vi "Modbus RT Driver VI Modbus.vi"(4 "DEBUG RT-FIFOs Indexes":T1[](array[typedef]), 6 "DEBUG General Settings":T3 {"Communication_Type" items=["TCP", "Serial"]; "Modbus_Type" items=["Master", "Slave"]; "Serial Settings"."Serial_Settings_Flow_Control" items=["None", "XONXOFF", "RTSCTS", "XONXOFFANDRTSCTS", "DTRDSR", "XONXOFFANDDTRDSR"]; "Serial Settings"."Serial_Settings_Parity" items=["None", "Odd", "Even"]; "Serial Settings"."Serial_Settings_Serial_Type" items=["RTU", "ASCII"]}, 7 "First FIFO Index of Status Channels":i32, 8 "error in (no error)":errorcluster, 9 "Inputs In":dbl[](array[numeric]), 10 "DEBUG Modbus Items":T9[](array[typedef]), 11 "Outputs In":dbl[](array[numeric])) -> (0 "error out":errorcluster, 3 "Outputs Out":dbl[](array[numeric]))   [LabVIEW 2014, in "Modbus Engine.lvlib"]
uses:
  Modbus Engine.lvlib
  XML Deserializer/XML VIs/API/Controls/Modbus_Items.ctl
  XML Deserializer/XML VIs/API/Controls/Modbus_Item_Type.ctl
  XML Deserializer/XML VIs/API/Controls/Modbus_General_Settings.ctl
  XML Deserializer/XML VIs/API/Controls/Modbus_Communication_Type.ctl
  XML Deserializer/XML VIs/API/Controls/Modbus_Type.ctl
  XML Deserializer/XML VIs/API/Controls/Modbus_Serial_Settings_Flow_Control.ctl
  XML Deserializer/XML VIs/API/Controls/Modbus_Serial_Settings_Parity.ctl
  XML Deserializer/XML VIs/API/Controls/Modbus_Serial_Settings_Serial_Type.ctl
  Shared/FIFO Indexes.ctl
  <vilib>/NI Veristand/Custom Device API/Custom Device Channel Type.ctl
  Modbus RT Driver VI States Definition.ctl
  ModbusPharLap.lvlibp/Modbus Library/API/Modbus API.lvclass
  <vilib>/NI Veristand/Custom Device Tools/Custom Device Utility Library/RT Debug String Color Spec.ctl
  Shared/Modbus Shared.lvlib
  ModbusPharLap.lvlibp/Modbus Library/API/Wrapper/API Main.lvlib
  <vilib>/NI Veristand/Custom Device Tools/Custom Device Utility Library/Custom Device Utility Library.lvlib
  ModbusPharLap.lvlibp/Modbus Library/API/Master/Modbus Master.lvclass
  <vilib>/NI Veristand/Custom Device API/Custom Device API.lvlib
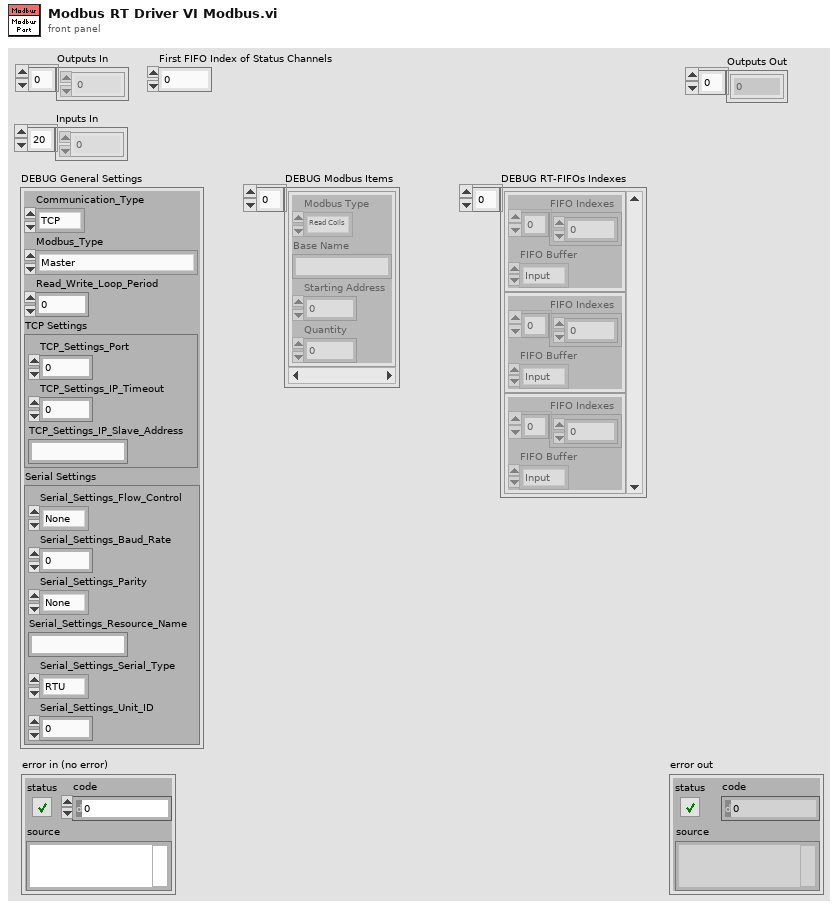
[diagram p1: front panel]
types:
  T1 = typedef "Modbus Shared.lvlib/FIFO Indexes.ctl" = cluster{"FIFO Indexes":i32[], "FIFO Buffer":T2}
  T2 = typedef "Custom Device API.lvlib/Custom Device Channel Type.ctl" = enum16{"Input", "Output"}
  T3 = typedef "Modbus Shared.lvlib/Modbus_General_Settings.ctl" = cluster{"Communication_Type":T4, "Modbus_Type":T5, "Read_Write_Loop_Period":i64, "TCP Settings":cluster{"TCP_Settings_Port":u16, "TCP_Settings_IP_Timeout":u32, "TCP_Settings_IP_Slave_Address":string}, "Serial Settings":cluster{"Serial_Settings_Flow_Control":T6, "Serial_Settings_Baud_Rate":u32, "Serial_Settings_Parity":T7, "Serial_Settings_Resource_Name":string, "Serial_Settings_Serial_Type":T8, "Serial_Settings_Unit_ID":u8}}
  T4 = typedef "Modbus Shared.lvlib/Modbus_Communication_Type.ctl" = i32
  T5 = typedef "Modbus Shared.lvlib/Modbus_Type.ctl" = i32
  T6 = typedef "Modbus Shared.lvlib/Modbus_Serial_Settings_Flow_Control.ctl" = i32
  T7 = typedef "Modbus Shared.lvlib/Modbus_Serial_Settings_Parity.ctl" = i32
  T8 = typedef "Modbus Shared.lvlib/Modbus_Serial_Settings_Serial_Type.ctl" = i32
  T9 = typedef "Modbus Shared.lvlib/Modbus_Items.ctl" = cluster{"Modbus Type":T10, "Base Name":string, "Starting Address":u16, "Quantity":u16}
  T10 = typedef "Modbus Shared.lvlib/Modbus_Item_Type.ctl" = enum16{"Read Coils", "Read Discrete Inputs", "Read Holding Registers", "Read Input Registers", "Write Multiple Coils", "Write Multiple Holding Registers", "Write Single Coil", "Write Single Holding Register", "Write Multiple Discrete Inputs", "Write Multiple Input Registers"}
  T11 = typedef "Modbus Engine.lvlib/Modbus RT Driver VI States Definition.ctl" = enum16{"Initialization", "Master - Connect", "Slave - Create Instance", "Exit", "Connected"}
  T12 = typedef "Custom Device Utility Library.lvlib/RT Debug String Color Spec.ctl" = u16
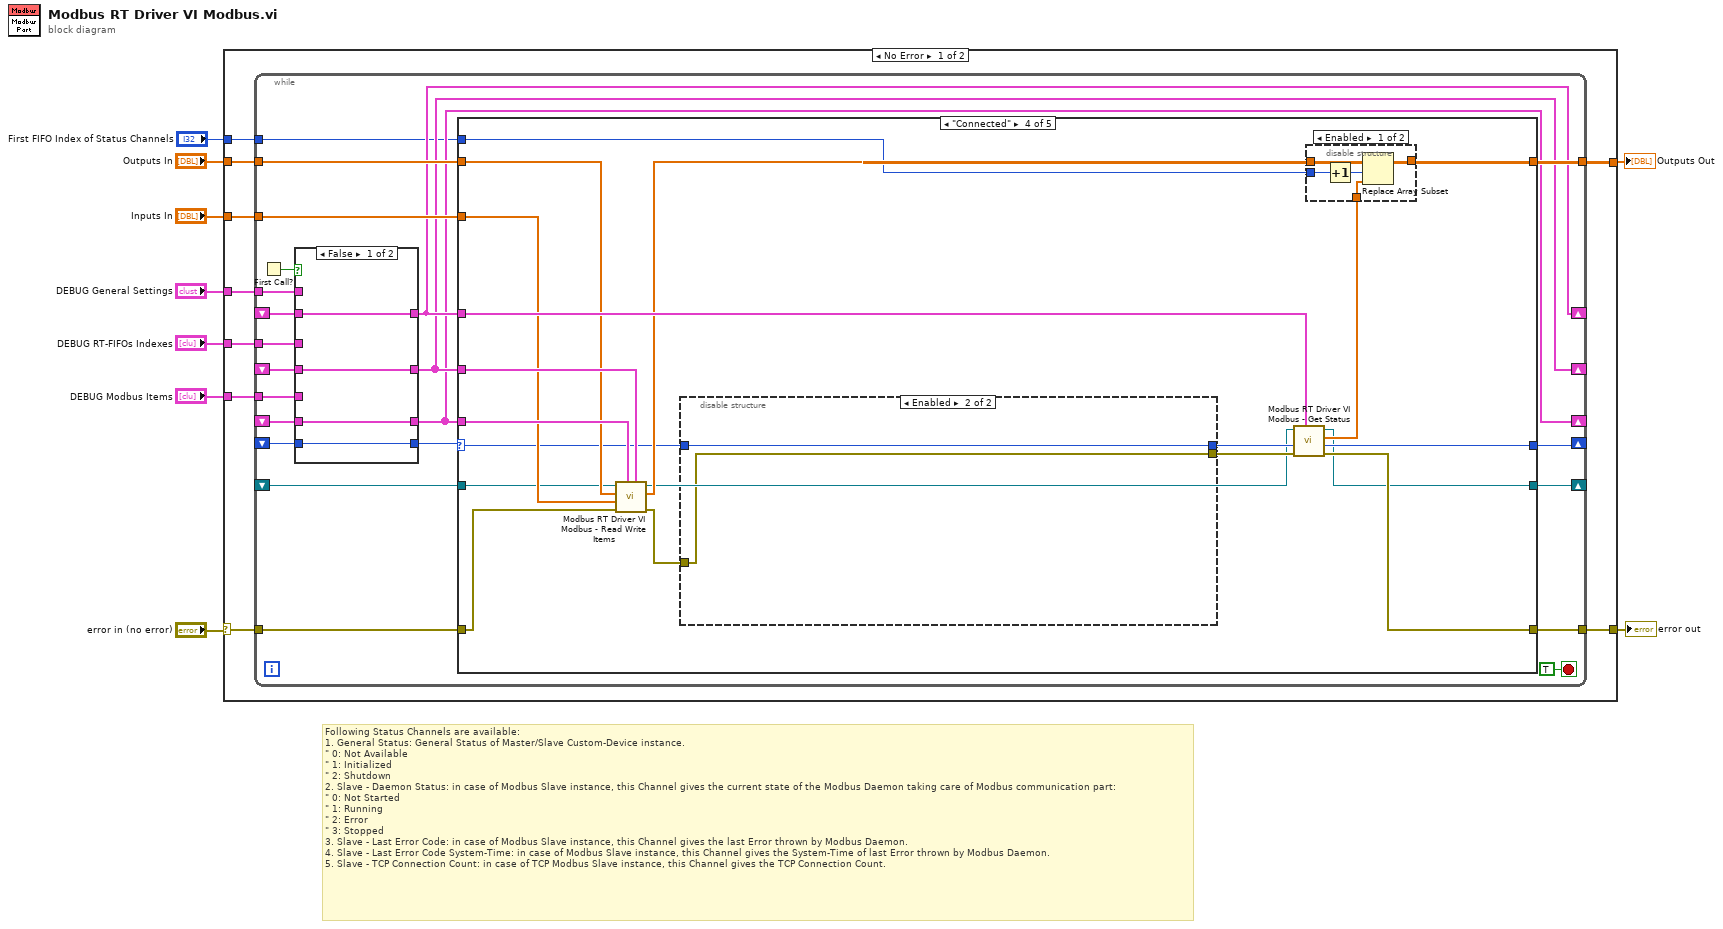
[diagram p0: block diagram]
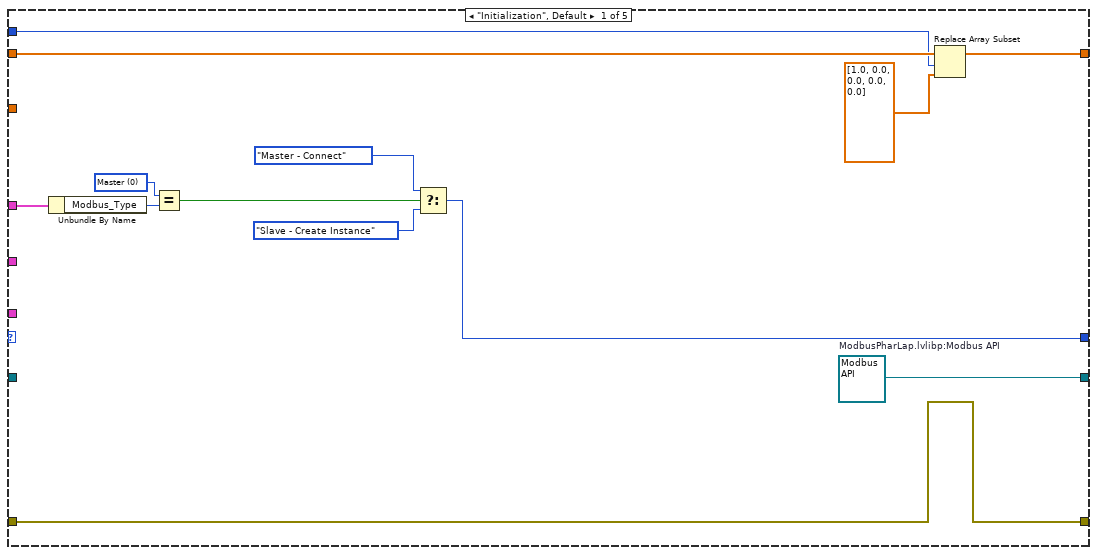
[diagram p2: hidden frame]
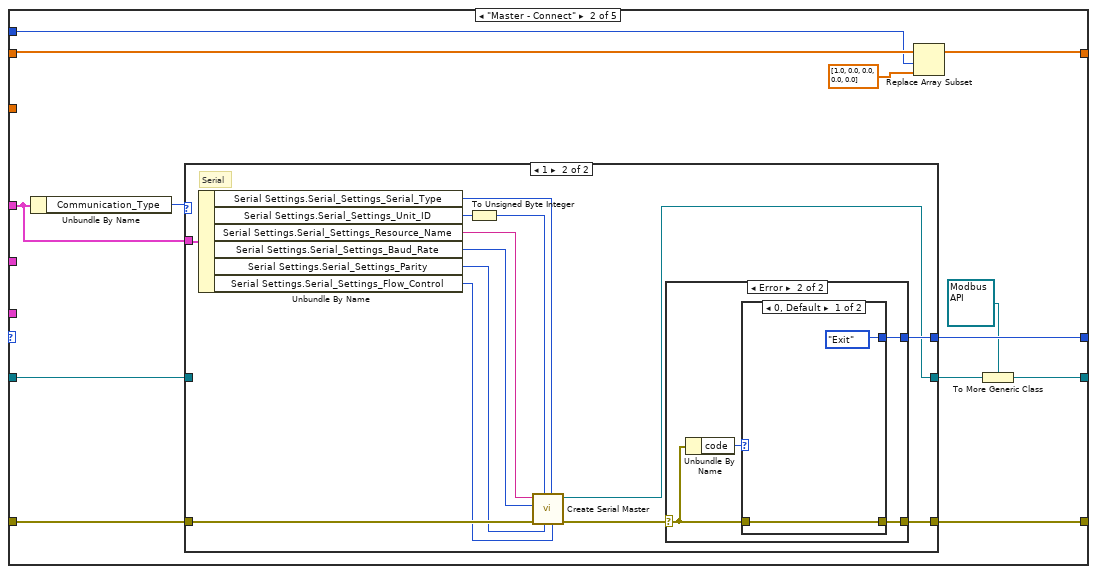
[diagram p3: hidden frame]
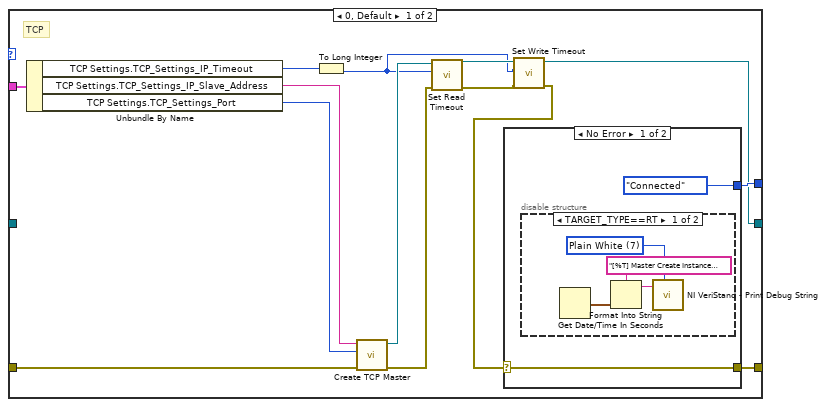
[diagram p4: hidden frame]
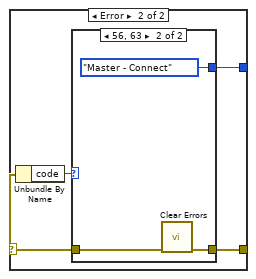
[diagram p6: hidden frame]
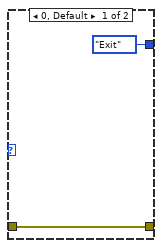
[diagram p7: hidden frame]
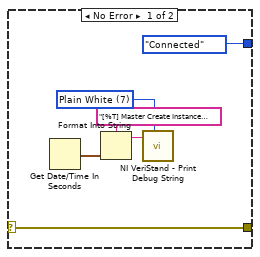
[diagram p8: hidden frame]
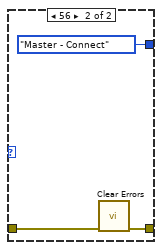
[diagram p9: hidden frame]
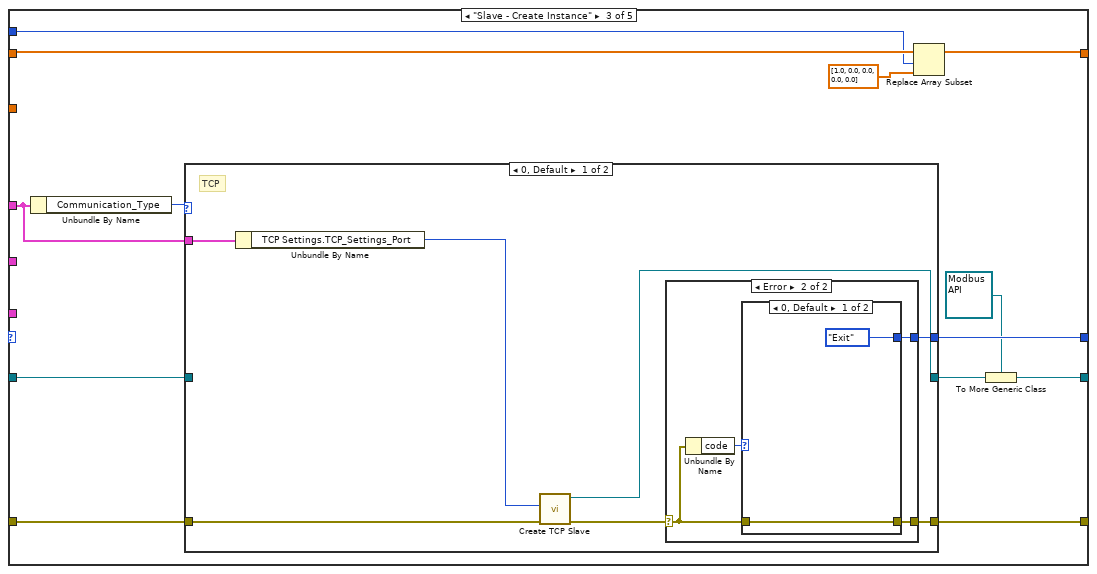
[diagram p10: hidden frame]
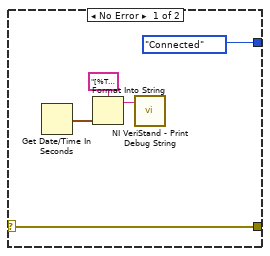
[diagram p11: hidden frame]
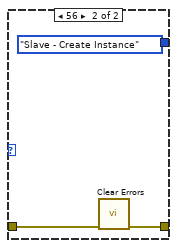
[diagram p12: hidden frame]
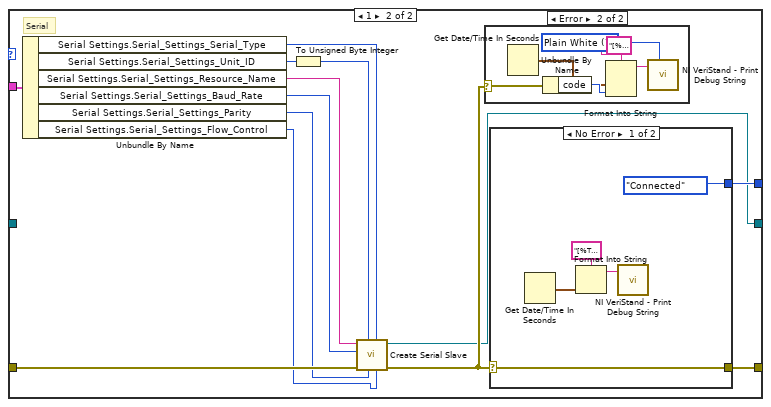
[diagram p13: hidden frame]
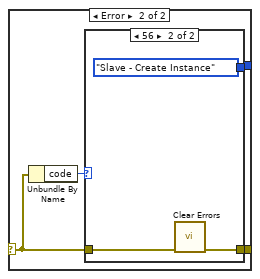
[diagram p15: hidden frame]
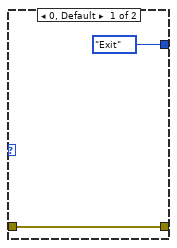
[diagram p16: hidden frame]
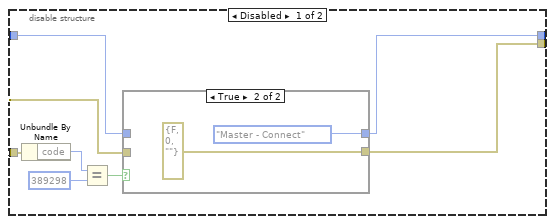
[diagram p17: hidden frame]
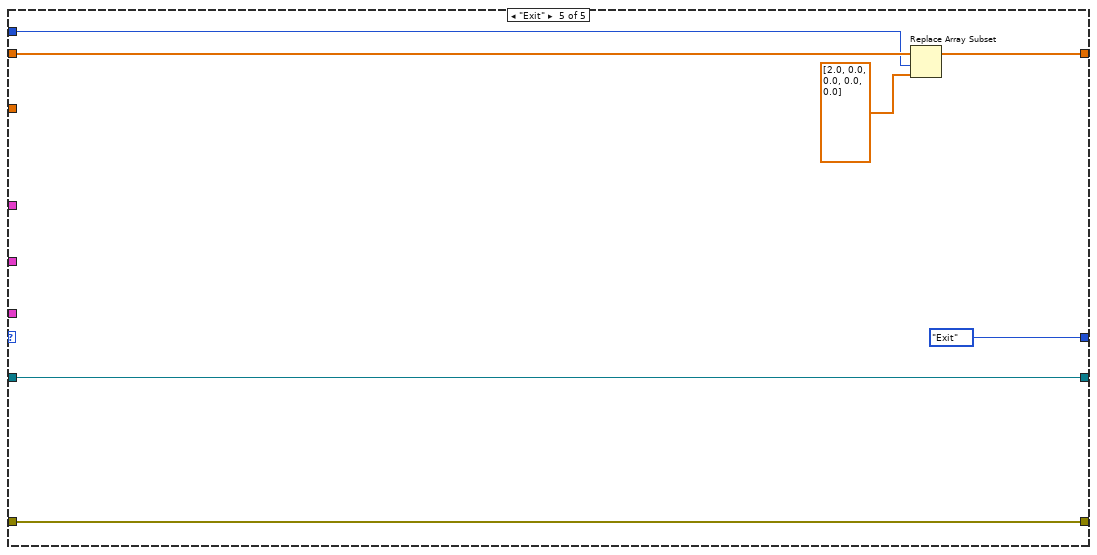
[diagram p20: hidden frame]
diagram:
  # "Following Status Channels are available:\n1. General Status: General Status of Master/Slave Custom-Device instance.\n\"\t0: Not Available\n\"\t1: Initialized\n\"\t2: Shutdown\n2. Slave - Daemon Status: in case of Modbus Slave instance, this Channel gives the current state of the Modbus Daemon taking care of Modbus communication part:\n\"\t0: Not Started\n\"\t1: Running\n\"\t2: Error\n\"\t3: Stopped\n3. Slave - Last Error Code: in case of Modbus Slave instance, this Channel gives the last Error thrown by Modbus Daemon.\n4. Slave - Last Error Code System-Time: in case of Modbus Slave instance, this Channel gives the System-Time of last Error thrown by Modbus Daemon.\n5. Slave - TCP Connection Count: in case of TCP Modbus Slave instance, this Channel gives the TCP Connection Count."
  n1 = case shown="No Error" "error in (no error)" {
    selector: "error in (no error)" -> [w18 w245]
    tunnel: [w17 w245] -> w8
    tunnel: "Outputs In" -> [w16 w244]
    tunnel: [w15 w244] -> w6
    tunnel: "Inputs In" -> [w14 _]
    tunnel: "DEBUG General Settings" -> [w13 _]
    tunnel: "DEBUG RT-FIFOs Indexes" -> [w12 _]
    tunnel: "DEBUG Modbus Items" -> [w11 _]
    tunnel: "First FIFO Index of Status Channels" -> [w10 _]
    frame No Error {
      n2 = while {
        tunnel: w18 -> [w23]
        tunnel: [w22] -> w17
        tunnel: w16 -> [w30]
        tunnel: [w29] -> w15
        tunnel: w14 -> [w31]
        shift-right: [w28] -> _
        shift-left: _ -> [w36]
        shift-right: [w27] -> _
        shift-left: _ -> [w35]
        shift-right: [w26] -> _
        shift-left: _ -> [w34]
        tunnel: w13 -> [w39]
        tunnel: w12 -> [w38]
        tunnel: w11 -> [w37]
        shift-right: [w25] -> _
        shift-left: _ -> [w24]
        shift-right: [w21] -> _
        shift-left: _ -> [w20]
        tunnel: w10 -> [w19]
        stop <- TRUE stop-if-true
        n3 = First Call?() -> (First Call?: T/F=w40:bool)
        n4 = case shown="False" w40 {
          tunnel: w39 -> [_ w243]
          tunnel: w38 -> [_ w242]
          tunnel: w37 -> [_ w241]
          tunnel: [w239 w243] -> w28
          tunnel: w36 -> [w239 _]
          tunnel: [w238 w242] -> w27
          tunnel: [w237 w241] -> w26
          tunnel: w35 -> [w238 _]
          tunnel: w34 -> [w237 _]
          tunnel: [w236 Modbus_RT_Driver_VI_States_Definition."Initialization"] -> w32
          tunnel: w24 -> [w236 _]
          frame False {
          }
          frame True {
          }
        }
        n5 = case shown="\"Connected\"" w32 {
          selector: w32 -> [_ _ _ w197 _]
          tunnel: w31 -> [_ _ _ w201 _]
          tunnel: w30 -> [w47 w59 w129 w202 w231]
          tunnel: [w46 w58 w128 w209 w230] -> w29
          tunnel: w28 -> [w53 w64 w134 w207 _]
          tunnel: w27 -> [_ _ _ w203 _]
          tunnel: w26 -> [_ _ _ w204 _]
          tunnel: [w48 w61 w131 w200 Modbus_RT_Driver_VI_States_Definition."Exit"] -> w25
          tunnel: w23 -> [w41 w63 w133 w205 w235]
          tunnel: [w41 w62 w132 w208 w235] -> w22
          tunnel: [w42 w55 w125 w192 w234] -> w21
          tunnel: w20 -> [_ w65 w135 w191 w234]
          tunnel: w19 -> [w43 w57 w127 w198 w229]
          frame "Initialization", Default {
            w42 = refnum<class "Modbus API.lvclass"> refnum  # ModbusPharLap.lvlibp:Modbus API
            w52 = T5 0 items=["Master", "Slave"] ("x")
            n6 = Unbundle By Name(w53) -> ("Modbus_Type"=w44:T5)
            n7 = Equal?(x=w52, y=w44) -> (x = y?=w51:bool)
            n8 = Select(t=Modbus_RT_Driver_VI_States_Definition."Master - Connect", s=w51, f=Modbus_RT_Driver_VI_States_Definition."Slave - Create Instance") -> (s? t:f=w48:T11)
            n9 = Replace Array Subset(array=w47, new element=dbl[] [1.0, 0.0, 0.0, 0.0, 0.0], index=w43) -> (w46:dbl[])
          }
          frame "Master - Connect" {
            n10 = Unbundle By Name(w64) -> ("Communication_Type"=w66:T4)
            n11 = case shown="1" w66 {
              tunnel: w65 -> [_ _]
              tunnel: w64 -> [w80 w107]
              tunnel: w63 -> [w75 w108]
              tunnel: [w76 w102] -> w62
              tunnel: [w68 w97] -> w56
              tunnel: [w77 w103] -> w61
              frame 0, Default {
                # "TCP"
                n12 = Unbundle By Name(w80) -> ("TCP Settings.TCP_Settings_IP_Timeout"=w74:u32, "TCP Settings.TCP_Settings_IP_Slave_Address"=w79:string, "TCP Settings.TCP_Settings_Port"=w78:u16)
                n13 = To Long Integer(number=w74) -> (32bit integer=w67:i32)
                n14 = call "Create TCP Master.vi"("error in"=w75, "port (502)"=w78, "address"=w79) -> ("error out"=w72:errorcluster, "TCP master instance"=w73:refnum<class "Modbus Master.lvclass">)  [unwired: 7 in]
                n15 = call "Set Read Timeout.vi"("error in"=w72, "read operation timeout"=w67, "Modbus master in"=w73) -> ("error out"=w71:errorcluster, "Modbus master out"=w69:refnum<class "Modbus Master.lvclass">)  [unwired: 7 in]
                n16 = call "Set Write Timeout.vi"("error in"=w71, "write operation timeout"=w67, "Modbus master in"=w69) -> ("error out"=w70:errorcluster, "Modbus master out"=w68:refnum<class "Modbus Master.lvclass">)  [unwired: 7 in]
                n17 = case shown="No Error" w70 {
                  selector: w70 -> [w81 w88]
                  tunnel: [Modbus_RT_Driver_VI_States_Definition."Connected" w89] -> w77
                  tunnel: [w81 w87] -> w76
                  frame No Error {
                    n18 = disable-structure shown="TARGET_TYPE==RT" {
                      frame condition #0 (active) {
                        w83 = T12 7 items=["Plain White"=7, "Bold White"=15, "Bold Blue"=9, "Bold Green"=10, "Bold Red"=12] ("Attribute")
                        n19 = Get Date/Time In Seconds() -> (seconds since 1Jan1904=w86:timestamp)
                        n20 = Format Into String(format string="[%T] Master Create Instance Succes.\n", w86) -> (resulting string=w84:string)  [unwired: 2 in, 1 out]
                        n21 = call <vilib>:"NI VeriStand - Print Debug String.vi"("Attribute"=w83, "Message"=w84) -> ()  [unwired: 9 in, 1 out]
                      }
                      frame condition #1 {
                      }
                    }
                  }
                  frame Error {
                    n22 = Unbundle By Name(w88) -> ("code"=w90:i32)
                    n23 = case shown="56, 63" w90 {
                      tunnel: [Modbus_RT_Driver_VI_States_Definition."Exit" Modbus_RT_Driver_VI_States_Definition."Master - Connect"] -> w89
                      tunnel: w88 -> [w91 w93]
                      tunnel: [w91 w94] -> w87
                      frame 0, Default {
                      }
                      frame 56, 63 {
                        n24 = call <vilib>:"Clear Errors.vi"("error in (no error)"=w93) -> ("error out"=w94:errorcluster)  [unwired: 5 in, 1 out]
                      }
                    }
                  }
                }
              }
              frame 1 {
                # "Serial"
                n25 = Unbundle By Name(w107) -> ("Serial Settings.Serial_Settings_Serial_Type"=w96:T8, "Serial Settings.Serial_Settings_Unit_ID"=w101:u8, "Serial Settings.Serial_Settings_Resource_Name"=w106:string, "Serial Settings.Serial_Settings_Baud_Rate"=w105:u32, "Serial Settings.Serial_Settings_Parity"=w98:T7, "Serial Settings.Serial_Settings_Flow_Control"=w99:T6)
                n26 = To Unsigned Byte Integer(number=w101) -> (unsigned 8bit integer=w100:u8)
                n27 = call "Create Serial Master.vi"("flow control (none)"=w99, "serial type"=w96, "parity (even)"=w98, "unit ID"=w100, "error in"=w108, "baud rate"=w105, "VISA resource name"=w106) -> ("error out"=w104:errorcluster, "serial master instance"=w97:refnum<class "Modbus Master.lvclass">)  [unwired: 3 in]
                n28 = case shown="Error" w104 {
                  selector: w104 -> [w113 w116]
                  tunnel: [Modbus_RT_Driver_VI_States_Definition."Connected" w117] -> w103
                  tunnel: [w113 w115] -> w102
                  frame No Error {
                    w109 = T12 7 items=["Plain White"=7, "Bold White"=15, "Bold Blue"=9, "Bold Green"=10, "Bold Red"=12] ("Attribute")
                    n29 = Get Date/Time In Seconds() -> (seconds since 1Jan1904=w112:timestamp)
                    n30 = Format Into String(format string="[%T] Master Create Instance Succes.\n", w112) -> (resulting string=w110:string)  [unwired: 2 in, 1 out]
                    n31 = call <vilib>:"NI VeriStand - Print Debug String.vi"("Attribute"=w109, "Message"=w110) -> ()  [unwired: 9 in, 1 out]
                  }
                  frame Error {
                    n32 = Unbundle By Name(w116) -> ("code"=w118:i32)
                    n33 = case shown="0, Default" w118 {
                      tunnel: [Modbus_RT_Driver_VI_States_Definition."Exit" Modbus_RT_Driver_VI_States_Definition."Master - Connect"] -> w117
                      tunnel: w116 -> [w119 w121]
                      tunnel: [w119 w122] -> w115
                      frame 0, Default {
                      }
                      frame 56 {
                        n34 = call <vilib>:"Clear Errors.vi"("error in (no error)"=w121) -> ("error out"=w122:errorcluster)  [unwired: 5 in, 1 out]
                      }
                    }
                  }
                }
              }
            }
            n35 = Replace Array Subset(array=w59, new element=dbl[] [1.0, 0.0, 0.0, 0.0, 0.0], index=w57) -> (w58:dbl[])
            n36 = To More Generic Class(target class=refnum<class "Modbus API.lvclass"> refnum ("ModbusPharLap.lvlibp:Modbus API"), reference=w56) -> (generic class reference=w55:refnum<class "Modbus API.lvclass">)
          }
          frame "Slave - Create Instance" {
            n37 = Unbundle By Name(w134) -> ("Communication_Type"=w136:T4)
            n38 = case shown="0, Default" w136 {
              tunnel: w135 -> [_ _]
              tunnel: w134 -> [w143 w169]
              tunnel: w133 -> [w138 w170]
              tunnel: [w141 w165] -> w132
              tunnel: [w139 w158] -> w126
              tunnel: [w142 w166] -> w131
              frame 0, Default {
                # "TCP"
                n39 = Unbundle By Name(w143) -> ("TCP Settings.TCP_Settings_Port"=w140:u16)
                n40 = call "Create TCP Slave.vi"("error in"=w138, "port (502)"=w140) -> ("error out"=w137:errorcluster, "TCP slave instance"=w139:refnum<class "Modbus Slave.lvclass">)  [unwired: 8 in]
                n41 = case shown="Error" w137 {
                  selector: w137 -> [w147 w150]
                  tunnel: [Modbus_RT_Driver_VI_States_Definition."Connected" w151] -> w142
                  tunnel: [w147 w149] -> w141
                  frame No Error {
                    n42 = Get Date/Time In Seconds() -> (seconds since 1Jan1904=w146:timestamp)
                    n43 = Format Into String(format string="[%T] Slave Create Instance Succes.\n", w146) -> (resulting string=w144:string)  [unwired: 2 in, 1 out]
                    n44 = call <vilib>:"NI VeriStand - Print Debug String.vi"("Message"=w144) -> ()  [unwired: 10 in, 1 out]
                  }
                  frame Error {
                    n45 = Unbundle By Name(w150) -> ("code"=w152:i32)
                    n46 = case shown="0, Default" w152 {
                      tunnel: [Modbus_RT_Driver_VI_States_Definition."Exit" Modbus_RT_Driver_VI_States_Definition."Slave - Create Instance"] -> w151
                      tunnel: w150 -> [w153 w155]
                      tunnel: [w153 w156] -> w149
                      frame 0, Default {
                      }
                      frame 56 {
                        n47 = call <vilib>:"Clear Errors.vi"("error in (no error)"=w155) -> ("error out"=w156:errorcluster)  [unwired: 5 in, 1 out]
                      }
                    }
                  }
                }
              }
              frame 1 {
                # "Serial"
                n48 = Unbundle By Name(w169) -> ("Serial Settings.Serial_Settings_Serial_Type"=w162:T8, "Serial Settings.Serial_Settings_Unit_ID"=w164:u8, "Serial Settings.Serial_Settings_Resource_Name"=w168:string, "Serial Settings.Serial_Settings_Baud_Rate"=w167:u32, "Serial Settings.Serial_Settings_Parity"=w160:T7, "Serial Settings.Serial_Settings_Flow_Control"=w161:T6)
                n49 = To Unsigned Byte Integer(number=w164) -> (unsigned 8bit integer=w163:u8)
                n50 = call "Create Serial Slave.vi"("flow control"=w161, "serial type"=w162, "parity (even)"=w160, "unit ID"=w163, "error in"=w170, "baud rate (9600)"=w167, "VISA resource name"=w168) -> ("error out"=w159:errorcluster, "serial slave instance"=w158:refnum<class "Modbus Slave.lvclass">)  [unwired: 3 in]
                n51 = case shown="Error" w159 {
                  selector: w159 -> [_ w176]
                  frame No Error {
                  }
                  frame Error {
                    w171 = T12 7 items=["Plain White"=7, "Bold White"=15, "Bold Blue"=9, "Bold Green"=10, "Bold Red"=12] ("Attribute")
                    n52 = Get Date/Time In Seconds() -> (seconds since 1Jan1904=w172:timestamp)
                    n53 = Unbundle By Name(w176) -> ("code"=w175:i32)
                    n54 = Format Into String(format string="[%T] Slave Create Instance Error: %d\n", w172, w175) -> (resulting string=w174:string)  [unwired: 2 in, 1 out]
                    n55 = call <vilib>:"NI VeriStand - Print Debug String.vi"("Attribute"=w171, "Message"=w174) -> ()  [unwired: 9 in, 1 out]
                  }
                }
                n56 = case shown="No Error" w159 {
                  selector: w159 -> [w180 w183]
                  tunnel: [Modbus_RT_Driver_VI_States_Definition."Connected" w184] -> w166
                  tunnel: [w180 w182] -> w165
                  frame No Error {
                    n57 = Get Date/Time In Seconds() -> (seconds since 1Jan1904=w179:timestamp)
                    n58 = Format Into String(format string="[%T] Slave Create Instance Succes.\n", w179) -> (resulting string=w177:string)  [unwired: 2 in, 1 out]
                    n59 = call <vilib>:"NI VeriStand - Print Debug String.vi"("Message"=w177) -> ()  [unwired: 10 in, 1 out]
                  }
                  frame Error {
                    n60 = Unbundle By Name(w183) -> ("code"=w185:i32)
                    n61 = case shown="56" w185 {
                      tunnel: [Modbus_RT_Driver_VI_States_Definition."Exit" Modbus_RT_Driver_VI_States_Definition."Slave - Create Instance"] -> w184
                      tunnel: w183 -> [w186 w188]
                      tunnel: [w186 w189] -> w182
                      frame 0, Default {
                      }
                      frame 56 {
                        n62 = call <vilib>:"Clear Errors.vi"("error in (no error)"=w188) -> ("error out"=w189:errorcluster)  [unwired: 5 in, 1 out]
                      }
                    }
                  }
                }
              }
            }
            n63 = Replace Array Subset(array=w129, new element=dbl[] [1.0, 0.0, 0.0, 0.0, 0.0], index=w127) -> (w128:dbl[])
            n64 = To More Generic Class(target class=refnum<class "Modbus API.lvclass"> refnum ("ModbusPharLap.lvlibp:Modbus API"), reference=w126) -> (generic class reference=w125:refnum<class "Modbus API.lvclass">)
          }
          frame "Connected" {
            n65 = call "Modbus RT Driver VI Modbus - Read Write Items.vi"("DEBUG RT-FIFOs Indexes"=w203, "DEBUG Modbus Items"=w204, "error in (no error)"=w205, "Inputs In"=w201, "Outputs In"=w202, "ModbusPharLap.lvlibp:Modbus API"=w191) -> ("error out"=w195:errorcluster, "Outputs Out"=w199:dbl[], "ModbusPharLap.lvlibp:Modbus API"=w193:refnum<class "Modbus API.lvclass">)  [unwired: 3 in]
            n66 = disable-structure shown="Enabled" {
              disable-tunnel: w197 -> [w216 w222]
              disable-tunnel: [w215 w222] -> w196
              disable-tunnel: w195 -> [w214 w221]
              disable-tunnel: [w213 w221] -> w194
              frame Disabled {
                n67 = Unbundle By Name(w214) -> ("code"=w212:i32)
                n68 = Equal?(x=w212, y=389298) -> (x = y?=w210:bool)
                n69 = case shown="True" w210 {
                  tunnel: w216 -> [w218 _]
                  tunnel: [w218 Modbus_RT_Driver_VI_States_Definition."Master - Connect"] -> w215
                  tunnel: w214 -> [w217 _]
                  tunnel: [w217 errorcluster {"status"=FALSE, "code"=0, "source"=""} ("error out")] -> w213
                  frame False {
                  }
                  frame True {
                  }
                }
              }
              frame Enabled {
              }
            }
            n70 = call "Modbus RT Driver VI Modbus - Get Status.vi"("DEBUG General Settings"=w207, "error in (no error)"=w194, "State In"=w196, "ModbusPharLap.lvlibp:Modbus API"=w193) -> ("error out"=w208:errorcluster, 1:w200:T11, "Array"=w206:dbl[], "ModbusPharLap.lvlibp:Modbus API"=w192:refnum<class "Modbus API.lvclass">)  [unwired: 4 in]
            n71 = disable-structure shown="Enabled" {
              disable-tunnel: [w227 w228] -> w209
              disable-tunnel: w206 -> [w226 _]
              disable-tunnel: w199 -> [w225 w228]
              disable-tunnel: w198 -> [w223 _]
              frame Enabled {
                n72 = Increment(x=w223) -> (x+1=w224:i32)
                n73 = Replace Array Subset(array=w225, new element=w226, index=w224) -> (w227:dbl[])
              }
              frame Disabled {
              }
            }
          }
          frame "Exit" {
            n74 = Replace Array Subset(array=w231, new element=dbl[] [2.0, 0.0, 0.0, 0.0, 0.0], index=w229) -> (w230:dbl[])
          }
        }
      }
    }
    frame Error {
    }
  }
  "Outputs Out" <- w6
  "error out" <- w8
